vi "Main.vi"(11 "Module Admin":refnum<class "Delacor_lib_QMH_Module Admin.lvclass">) -> ()   [LabVIEW 2020, in "UI.lvlib"]
doc: "This template is based off of the Queued Message Handler design pattern and the Queued Message Handler project template that ships with LabVIEW.\n\nThe main difference is that the queue is private to this module and communication between modules is performed via Broadcast and Request events.\n\nRequest events are wrapped in public API methods and are handled in the Event Handling Loop (EHL) of this VI. Any module can register for Broadcast events sent by this module. The EHL generates messages based on user interface actions.\n\nThe Message Handling Loop (MHL) processes messages generated by the EHL, or by other messages. The messages are string values, so new messages can be added easily to the Message Cases case structure in the MHL. Each message cluster can also provide an optional value for Message Data, which is a variant that can be converted to whatever message-specific data is required.\n_____\nBased on Delacor QMH Project Template 5.0.0.82."
uses:
  UI.lvlib
  <vilib>/Delacor/Delacor QMH/Libraries/Module Admin_class/Delacor_lib_QMH_Module Admin.lvclass
  Module Data--cluster.ctl
  Stop Argument--cluster.ctl
  <vilib>/Delacor/Delacor QMH/Libraries/Message Queue_class/Delacor_lib_QMH_Message Queue.lvclass/Delacor_lib_QMH_Message Queue.ctl
  <vilib>/Utility/miscctls.llb/LVPointTypeDef.ctl
  <vilib>/Delacor/Delacor QMH/Libraries/Module Admin_class/Delacor_lib_QMH_Module Admin.lvclass/Delacor_lib_QMH_Module Admin.ctl
  <vilib>/Delacor/Delacor QMH/Libraries/Message Queue_class/Delacor_lib_QMH_Enqueue Message (Single).vi
  <vilib>/Delacor/Delacor QMH/Libraries/Module Admin_class/Delacor_lib_QMH_Get External Launch.vi
  <vilib>/Utility/error.llb/Error Cluster From Error Code.vi
  <vilib>/ErrorRing/Error Ring.xnode
  <vilib>/Delacor/Delacor QMH/Libraries/Message Queue_class/Delacor_lib_QMH_Message Queue.lvclass
  Acquisition/Acquisition.lvlib
  Config/Config.lvlib
  Loggin/Loggin.lvlib
panel:
  in  "Config":bool
  in  "Stop Acq":bool
  in  "Start Acq":bool
  out "error out":errorcluster
  out "Status":string
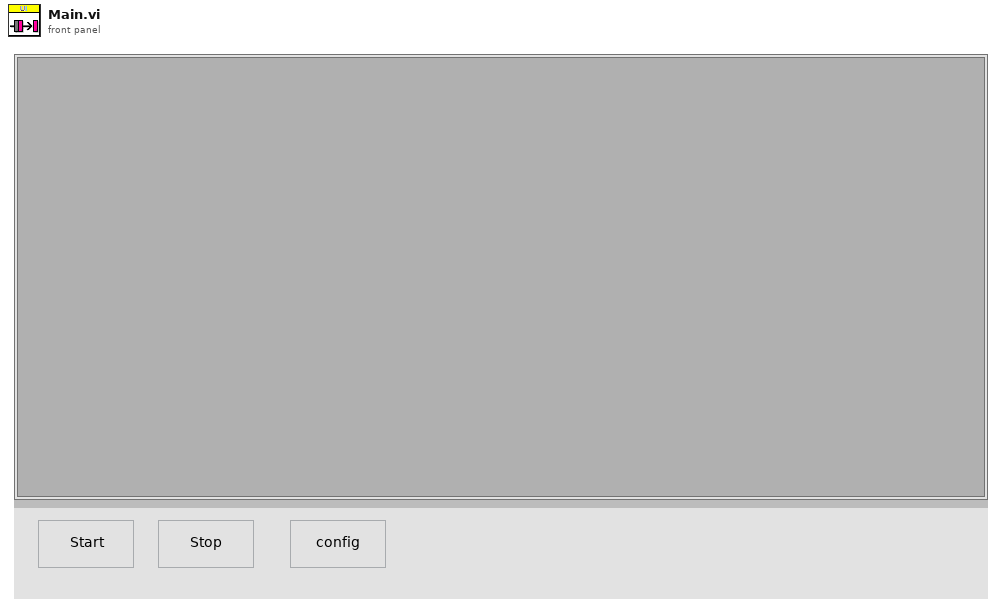
[diagram p1: front panel]
types:
  T1 = typedef "UI.lvlib/Request Events--cluster.ctl" = cluster{"Stop Module":refnum<user-event>, "Show Panel":refnum<user-event>, "Hide Panel":refnum<user-event>, "Get Module Execution Status":refnum<user-event>, "Show Diagram":refnum<user-event>}
  T2 = typedef "Config.lvlib/Broadcast Events--cluster.ctl" = cluster{"Module Did Init":refnum<user-event>, "Status Updated":refnum<user-event>, "Error Reported":refnum<user-event>, "Module Did Stop":refnum<user-event>, "Update Module Execution Status":refnum<user-event>}
  T3 = typedef "Acquisition.lvlib/Broadcast Events--cluster.ctl" = cluster{"Module Did Init":refnum<user-event>, "Status Updated":refnum<user-event>, "Error Reported":refnum<user-event>, "Module Did Stop":refnum<user-event>, "Update Module Execution Status":refnum<user-event>}
  T4 = typedef "Loggin.lvlib/Broadcast Events--cluster.ctl" = cluster{"Module Did Init":refnum<user-event>, "Status Updated":refnum<user-event>, "Error Reported":refnum<user-event>, "Module Did Stop":refnum<user-event>, "Update Module Execution Status":refnum<user-event>}
  T5 = typedef "UI.lvlib/Module Data--cluster.ctl" = cluster{"Status":string}
  T6 = enum32{"invalid lock state", "Not Locked", "Locked (No Password)", "Password-protected"}
  T7 = typedef "UI.lvlib/Stop Argument--cluster.ctl" = cluster{"Origin":string, "Exit via Stop Module Req?":bool, "Wait for Module to stop?":bool}
  T8 = enum32{"Invalid", "Standard", "Closed", "Hidden", "Minimized", "Maximized"}
  T9 = typedef "LVPointTypeDef.ctl" = cluster{"Horizontal":i16, "Vertical":i16}
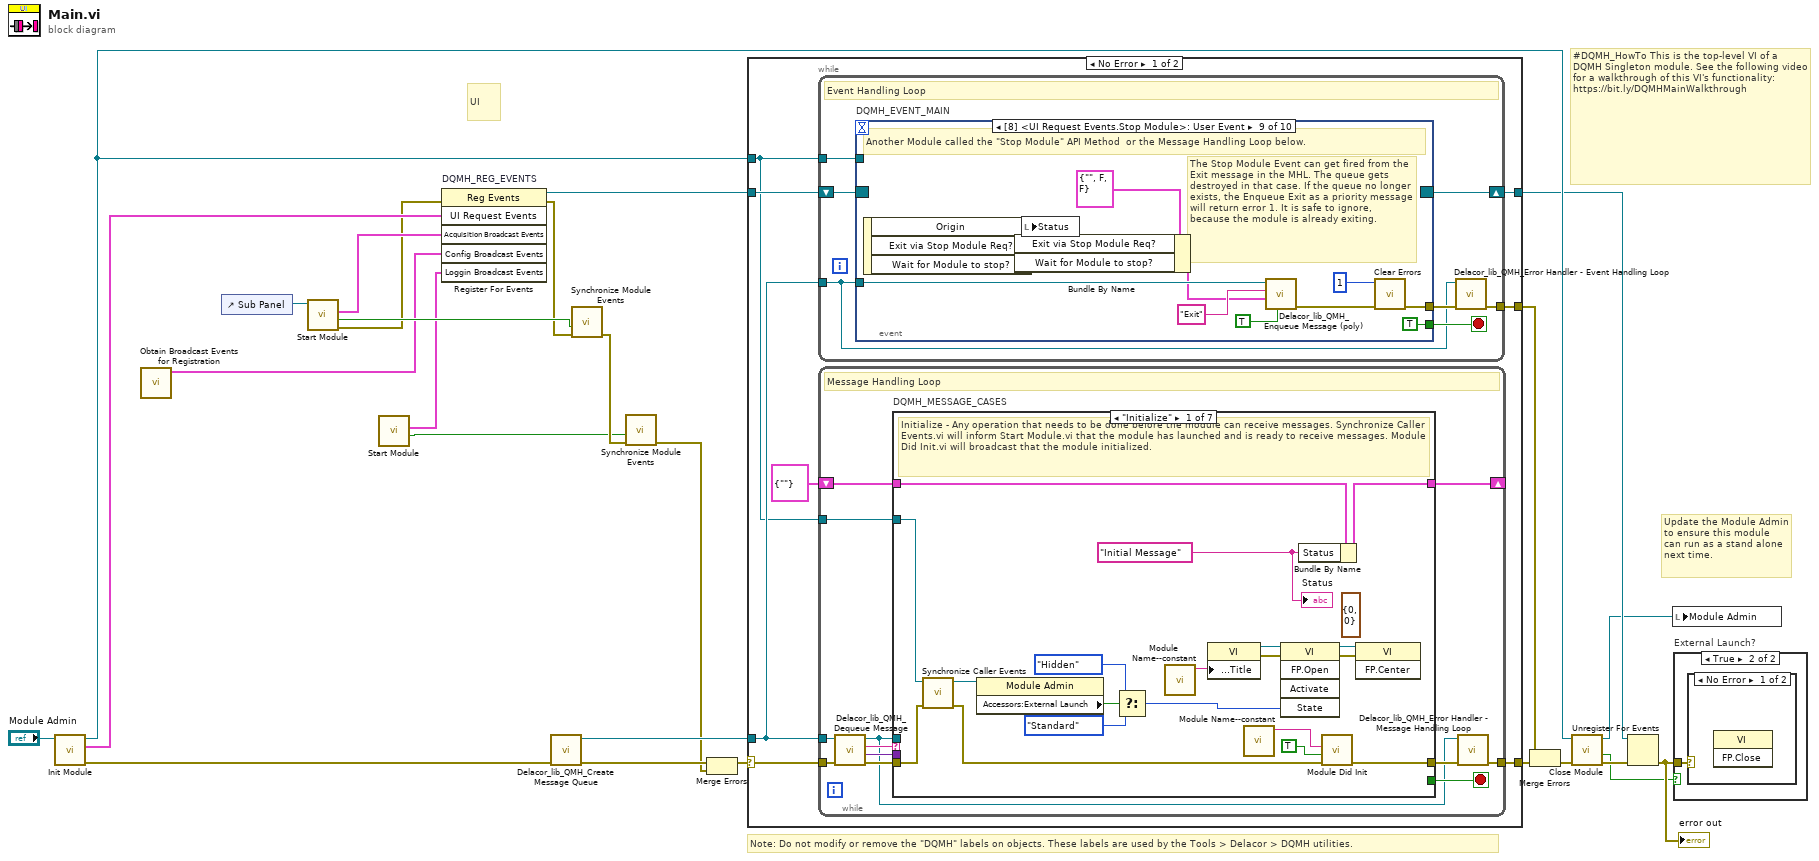
[diagram p0: block diagram]
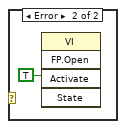
[diagram p3: hidden frame]
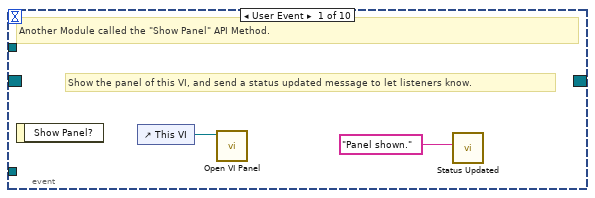
[diagram p4: hidden frame]
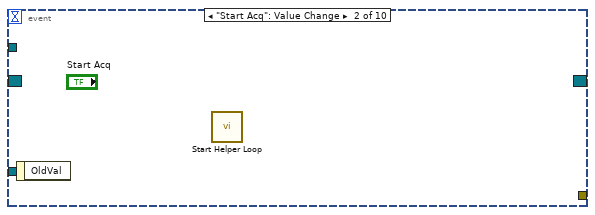
[diagram p5: hidden frame]
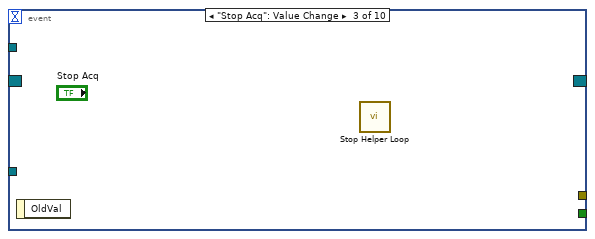
[diagram p6: hidden frame]
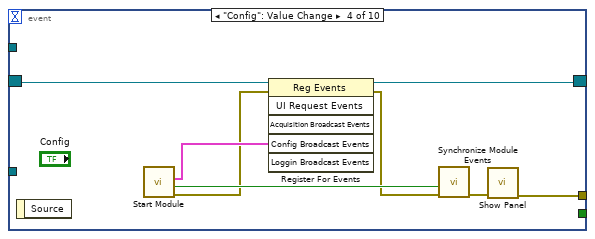
[diagram p7: hidden frame]
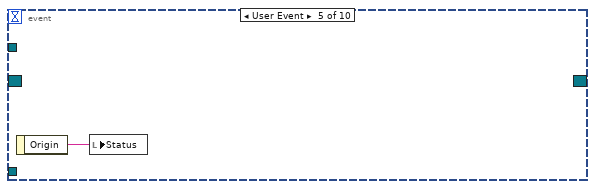
[diagram p8: hidden frame]
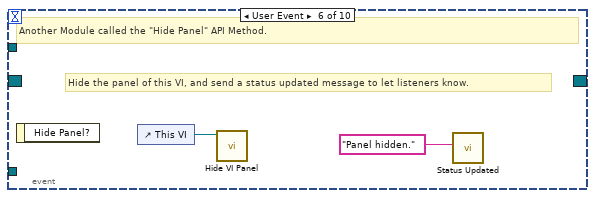
[diagram p9: hidden frame]
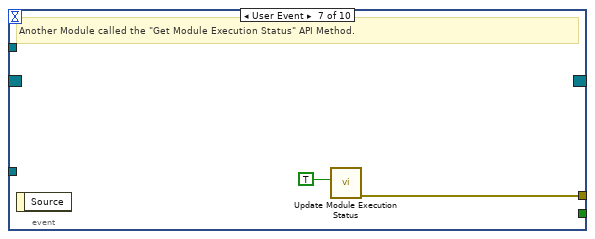
[diagram p10: hidden frame]
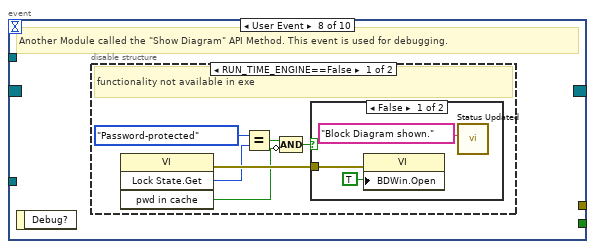
[diagram p11: hidden frame]
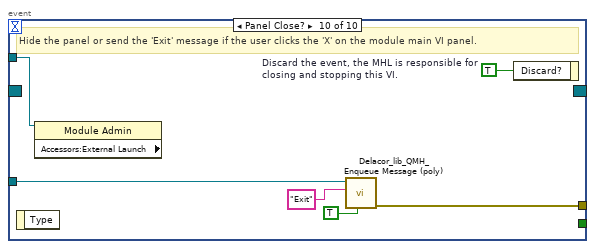
[diagram p14: hidden frame]
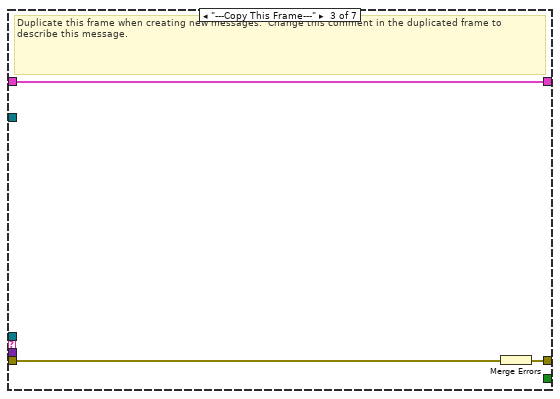
[diagram p16: hidden frame]
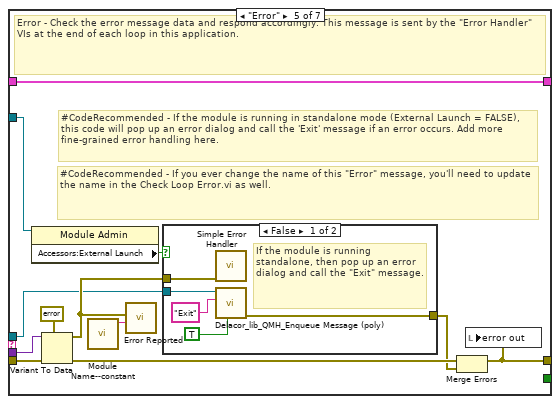
[diagram p18: hidden frame]
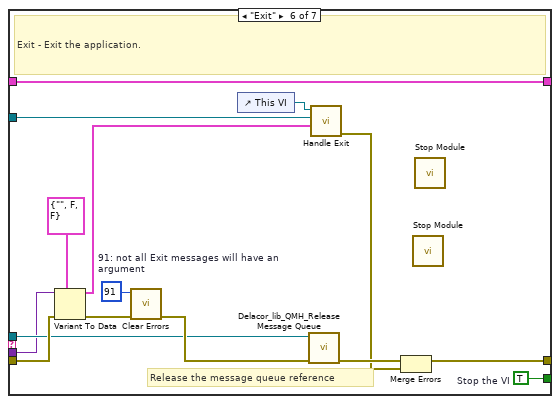
[diagram p20: hidden frame]
diagram:
  # "UI"
  # "#DQMH_HowTo This is the top-level VI of a DQMH Singleton module. See the following video for a walkthrough of this VI's functionality: https://bit.ly/DQMHMainWalkthrough"
  # "Note: Do not modify or remove the \"DQMH\" labels on objects. These labels are used by the Tools > Delacor > DQMH utilities."
  # "Update the Module Admin to ensure this module can run as a stand alone next time."
  n1 = call "Init Module.vi"("Singleton Module Admin in"="Module Admin") -> ("error out"=w25:errorcluster, "UI Request Events"=w15:T1, "Singleton Module Admin out"=w18:refnum<class "Delacor_lib_QMH_Module Admin.lvclass">)  [unwired: 8 in]
  n2 = call "Obtain Broadcast Events for Registration.vi"() -> ("Config Broadcast Events"=w5:T2)  [unwired: 9 in, 2 out]
  n3 = control-ref of="Sub Panel"() -> (w6:refnum<vi>)
  n4 = call "Start Module.vi"("Sub Panel"=w6) -> ("error out"=w7:errorcluster, "Wait for Event Sync?"=w9:bool, "Acquisition Broadcast Events"=w10:T3)  [unwired: 7 in, 1 out]
  n5 = call "Start Module.vi"() -> ("Wait for Event Sync?"=w2:bool, "Loggin Broadcast Events"=w1:T4)  [unwired: 8 in, 2 out]
  n6 = register-events "DQMH_REG_EVENTS"(error in=w7, w15, w10, w5, w1) -> (reference out=w16:refnum<event-registration>, error out=w8:errorcluster)  [unwired: 1 in]
  n7 = call <vilib>:"Delacor_lib_QMH_Create Message Queue.vi"("error in (no error)"=w25) -> ("error out"=w20:errorcluster, "Message Queue"=w14:refnum<class "Delacor_lib_QMH_Message Queue.lvclass">)  [unwired: 9 in]
  n8 = call "Synchronize Module Events.vi"("error in (no error)"=w8, "Wait for Event Sync?"=w9) -> ("error out"=w4:errorcluster)  [unwired: 9 in]
  n9 = call "Synchronize Module Events.vi"("error in (no error)"=w4, "Wait for Event Sync?"=w2) -> ("error out"=w3:errorcluster)  [unwired: 9 in]
  n10 = Merge Errors(w20, w3) -> (w19:errorcluster)
  n11 = case shown="No Error" w19 {
    selector: w19 -> [w32 w170]
    tunnel: [w34 w169] -> w26
    tunnel: [w31 w175] -> w17
    tunnel: w16 -> [w29 w175]
    tunnel: w14 -> [w28 w168]
    tunnel: [w33 _] -> w23
    tunnel: w18 -> [w27 w171]
    frame No Error {
      n12 = while {
        tunnel: w28 -> [w35]
        shift-right: [w38] -> w31
        shift-left: w29 -> [w39]
        tunnel: [w40] -> w33
        tunnel: w27 -> [w36]
        stop <- w37 stop-if-true
        # "Event Handling Loop"
        n13 = event "DQMH_EVENT_MAIN" shown="[8] <UI Request Events.Stop Module>: User Event" {
          selector: w39 -> [_ _ _ w51 _ _ _ _ _ _]
          dyn-events: [_ _ _ w50 _ _ _ _ _ _] -> w38
          timeout: _ -> [_ _ _ _ _ _ _ _ _ _]
          tunnel: [_ _ _ _ _ _ _ _ TRUE ("Discard?") _] -> w37
          tunnel: w35 -> [_ _ _ _ _ _ _ _ w73 w81]
          tunnel: [_ _ _ w44 _ _ w56 _ w76 w83] -> w41
          tunnel: w36 -> [_ _ _ _ _ _ _ _ _ w80]
          event User Event {
            # "Show the panel of this VI, and send a status updated message to let listeners know."
            # "Another Module called the \"Show Panel\" API Method."
            n14 = event-data() -> ()  [unwired: 1 in, 1 out]
            n15 = control-ref of="This VI"() -> (w43:refnum<vi>)
            n16 = call "Open VI Panel.vi"("VI"=w43) -> ()  [unwired: 10 in, 1 out]
            n17 = call "Status Updated.vi"("Status"="Panel shown." ("format string")) -> ()  [unwired: 10 in, 1 out]
          }
          event "Start Acq": Value Change {
            n18 = event-data() -> ()  [unwired: 1 in, 1 out]
            n19 = call "Start Helper Loop.vi"() -> ()  [unwired: 11 in, 1 out]
          }
          event "Stop Acq": Value Change {
            n20 = event-data() -> ()  [unwired: 1 in, 1 out]
            n21 = call "Stop Helper Loop.vi"() -> ()  [unwired: 11 in, 1 out]
          }
          event "Config": Value Change {
            n22 = event-data() -> ()  [unwired: 1 in, 1 out]
            n23 = call "Start Module.vi"() -> ("error out"=w47:errorcluster, "Wait for Event Sync?"=w48:bool, "Config Broadcast Events"=w49:T2)  [unwired: 8 in, 1 out]
            n24 = register-events(reference=w51, error in=w47, w49) -> (reference out=w50:refnum<event-registration>, error out=w46:errorcluster)  [unwired: 3 in]
            n25 = call "Synchronize Module Events.vi"("error in (no error)"=w46, "Wait for Event Sync?"=w48) -> ("error out"=w45:errorcluster)  [unwired: 9 in]
            n26 = call "Show Panel.vi"("error in (no error)"=w45) -> ("error out"=w44:errorcluster)  [unwired: 10 in]
          }
          event User Event {
            n27 = event-data() -> ("Origin"=w52:string)  [unwired: 1 in]
            n28 = local write "Status"(w52) -> ()
          }
          event User Event {
            # "Hide the panel of this VI, and send a status updated message to let listeners know."
            # "Another Module called the \"Hide Panel\" API Method."
            n29 = event-data() -> ()  [unwired: 1 in, 1 out]
            n30 = control-ref of="This VI"() -> (w54:refnum<vi>)
            n31 = call "Hide VI Panel.vi"("VI"=w54) -> ()  [unwired: 10 in, 1 out]
            n32 = call "Status Updated.vi"("Status"="Panel hidden." ("format string")) -> ()  [unwired: 10 in, 1 out]
          }
          event User Event {
            # "Another Module called the \"Get Module Execution Status\" API Method."
            n33 = event-data() -> ()  [unwired: 1 in, 1 out]
            n34 = call "Update Module Execution Status.vi"("Running?"=TRUE) -> ("error out"=w56:errorcluster)  [unwired: 10 in]
          }
          event User Event {
            # "Another Module called the \"Show Diagram\" API Method. This event is used for debugging."
            n35 = event-data() -> ()  [unwired: 1 in, 1 out]
            n36 = disable-structure shown="RUN_TIME_ENGINE==False" {
              frame condition #0 (active) {
                # "functionality not available in exe"
                n37 = invoke class="VI" method="Lock State.Get"() -> (error out=w62:errorcluster, "Get Lock State"=w61:T6, "pwd in cache"=w58:bool)  [unwired: 4 in, 1 out]
                n38 = Equal?(x=T6."Password-protected", y=w61) -> (x = y?=w59:bool)
                n39 = Compound Arithmetic op=AND(w59, invert w58) -> (w57:bool)
                n40 = case shown="False" w57 {
                  tunnel: w62 -> [w65 _]
                  frame False {
                    n41 = property class="VI"(error in=w65, "BDWin.Open"=TRUE ("Block Diagram Window:Open")) -> ()  [unwired: 1 in, 2 out]
                    n42 = call "Status Updated.vi"("Status"="Block Diagram shown." ("format string")) -> ()  [unwired: 10 in, 1 out]
                  }
                  frame True {
                    # "Password-protected VI, and the password is not in the cache. Do not show the diagram."
                  }
                }
              }
              frame condition #1 {
              }
            }
          }
          event User Event {
            # "The Stop Module Event can get fired from the Exit message in the MHL. The queue gets destroyed in that case. If the queue no longer exists, the Enqueue Exit as a priority message will return error 1. It is safe to ignore, because the module is already exiting."
            # "Another Module called the \"Stop Module\" API Method  or the Message Handling Loop below."
            n43 = event-data() -> ("Origin"=w72:string, "Exit via Stop Module Req?"=w68:bool, "Wait for Module to stop?"=w67:bool)  [unwired: 1 in]
            n44 = Bundle By Name(cluster=T7 {"Origin"="", "Exit via Stop Module Req?"=FALSE, "Wait for Module to stop?"=FALSE} ("Stop Argument"), "Exit via Stop Module Req?"=w68, "Wait for Module to stop?"=w67) -> (w66:T7)
            n45 = local write "Status"(w72) -> ()
            n46 = call-poly <vilib>:"Delacor_lib_QMH_Enqueue Message (poly).vi"("Priority Message? (F)"=TRUE, "Message Data"=w66, "Message"="Exit", "Message Queue in"=w73) -> ("error out"=w77:errorcluster)  [unwired: 6 in, 1 out]
            n47 = call <vilib>:"Clear Errors.vi"("error in (no error)"=w77, "specific error code to clear (0: all)"=1) -> ("error out"=w76:errorcluster)  [unwired: 4 in, 1 out]
          }
          event Panel Close? {
            w82 = TRUE  # Discard the event, the MHL is responsible for closing and stopping this VI.
            # "Hide the panel or send the 'Exit' message if the user clicks the 'X' on the module main VI panel."
            n48 = event-data() -> ()  [unwired: 1 in, 1 out]
            n49 = property class="Module Admin" props=["Accessors:External Launch"](reference=w80) -> ()  [unwired: 1 in, 3 out]
            n50 = call-poly <vilib>:"Delacor_lib_QMH_Enqueue Message (poly).vi"("Priority Message? (F)"=TRUE, "Message"="Exit", "Message Queue in"=w81) -> ("error out"=w83:errorcluster)  [unwired: 7 in, 1 out]
            n51 = event-data("Discard?"=w82) -> ()  [unwired: 1 in, 1 out]
          }
        }
        n52 = call-dynamic "Delacor_lib_QMH_Error Handler - Event Handling Loop.vi"("error in (no error)"=w41, "Message Queue in"=w35) -> ("dup error in"=w40:errorcluster)  [unwired: 8 in, 1 out]
      }
      n53 = while {
        tunnel: w28 -> [w86]
        shift-right: [w90] -> _
        shift-left: T5 {"Status"=""} ("Data Cluster") -> [w91]
        tunnel: w32 -> [w94]
        tunnel: [w92] -> w34
        tunnel: w27 -> [w84]
        stop <- w89 stop-if-true
        # "Message Handling Loop"
        n54 = call-dynamic "Delacor_lib_QMH_Dequeue Message.vi"("error in (no error)"=w94, "Message Queue in"=w86) -> ("error out"=w93:errorcluster, "Message Data"=w87:variant, "Message"=w88:string, "Message Queue out"=w85:refnum<class "Delacor_lib_QMH_Message Queue.lvclass">)  [unwired: 6 in]
        n55 = case "DQMH_MESSAGE_CASES" shown="\"Initialize\"" w88 {
          selector: w88 -> [_ _ _ _ _ _ w155]
          tunnel: w85 -> [_ _ _ _ w125 w147 _]
          tunnel: w93 -> [w112 w116 w119 w121 w132 w153 w157]
          tunnel: [w110 w116 w118 w121 w128 w150 w158] -> w95
          tunnel: w91 -> [w101 w115 w117 w120 w127 w146 w156]
          tunnel: [w100 w115 w117 w120 w127 w146 w156] -> w90
          tunnel: [_ _ _ _ _ w145 _] -> w89
          tunnel: w87 -> [_ _ _ _ w126 w144 _]
          tunnel: w84 -> [w102 _ _ _ w124 w139 _]
          frame "Initialize" {
            (unwired) T9 {"Horizontal"=0, "Vertical"=0} ("Origin")
            w96 = "Initial Message" ("Initial Message")
            # "Initialize - Any operation that needs to be done before the module can receive messages. Synchronize Caller Events.vi will inform Start Module.vi that the module has launched and is ready to receive messages. Module Did Init.vi will broadcast that the module initialized."
            n56 = call "Synchronize Caller Events.vi"("error in (no error)"=w112, "Singleton Module Admin in"=w102) -> ("error out"=w111:errorcluster, "Singleton Module Admin out"=w97:refnum<class "Delacor_lib_QMH_Module Admin.lvclass">)  [unwired: 8 in]
            n57 = property class="Module Admin"(reference=w97) -> ("Accessors:External Launch"=w106:bool)  [unwired: 1 in, 2 out]
            n58 = Select(t=T8."Hidden" ("State"), s=w106, f=T8."Standard" ("State")) -> (s? t:f=w103:T8)
            n59 = call "Module Name--constant.vi"() -> ("Module Name"=w109:string)  [unwired: 11 in]
            n60 = property class="VI"("Front Panel.Title"=w109) -> (reference out=w108:refnum<vi>, error out=w114:errorcluster)  [unwired: 2 in]
            n61 = call "Module Name--constant.vi"() -> ("Module Name"=w98:string)  [unwired: 11 in]
            n62 = invoke class="VI" method="FP.Open"(reference=w108, error in=w114, "State"=w103) -> (reference out=w107:refnum<vi>, error out=w113:errorcluster)  [unwired: 2 in, 3 out]
            n63 = Bundle By Name(cluster=w101, "Status"=w96) -> (w100:T5)
            n64 = call "Module Did Init.vi"("error in (no error)"=w111, "Initialized?"=TRUE, "Origin"=w98) -> ("error out"=w110:errorcluster)  [unwired: 8 in]
            n65 = invoke class="VI" method="FP.Center"(reference=w107, error in=w113) -> ()  [unwired: 1 in, 3 out]
            "Status" <- w96
          }
          frame "--- Module Specific ---" {
            # "Separator -- The following cases handle messages specific to this Module."
          }
          frame "---Copy This Frame---" {
            # "Duplicate this frame when creating new messages.  Change this comment in the duplicated frame to describe this message."
            n66 = Merge Errors(w119) -> (w118:errorcluster)
          }
          frame "--- Exit and Error Handling---" {
            # "Separator - The following cases handle errors and exit messages."
          }
          frame "Error" {
            # "#CodeRecommended - If you ever change the name of this \"Error\" message, you'll need to update the name in the Check Loop Error.vi as well."
            # "#CodeRecommended - If the module is running in standalone mode (External Launch = FALSE), this code will pop up an error dialog and call the 'Exit' message if an error occurs. Add more fine-grained error handling here."
            # "Error - Check the error message data and respond accordingly. This message is sent by the \"Error Handler\" VIs at the end of each loop in this application."
            n67 = property class="Module Admin"(reference=w124) -> ("Accessors:External Launch"=w123:bool)  [unwired: 1 in, 2 out]
            n68 = Variant To Data(error in=w132, type=errorcluster {"status"=FALSE, "code"=0, "source"=""} ("error constant"), Variant=w126) -> (data=w133:errorcluster, error out=w130:errorcluster)
            n69 = call "Module Name--constant.vi"() -> ("Module Name"=w122:string)  [unwired: 11 in]
            n70 = call "Error Reported.vi"("Additional Information"=w122, "Error"=w133) -> ()  [unwired: 9 in, 1 out]
            n71 = case shown="False" w123 {
              tunnel: [w138 _] -> w129
              tunnel: w125 -> [w136 _]
              tunnel: w133 -> [w137 _]
              frame False {
                # "If the module is running standalone, then pop up an error dialog and call the \"Exit\" message."
                n72 = call <vilib>:"Simple Error Handler.vi"("error in (no error)"=w137) -> ()  [unwired: 4 in, 5 out]
                n73 = call-poly <vilib>:"Delacor_lib_QMH_Enqueue Message (poly).vi"("Priority Message? (F)"=TRUE, "Message"="Exit", "Message Queue in"=w136) -> ("error out"=w138:errorcluster)  [unwired: 7 in, 1 out]
              }
              frame True {
                # "If the module was launched externally, calling the Error Reported broadcast VI is the only action performed by the \"Error\" message. The module's caller can then process the error appropriately."
              }
            }
            n74 = Merge Errors(w130, w129) -> (w128:errorcluster)
            n75 = local write "error out"(w128) -> ()
          }
          frame "Exit" {
            w143 = 91  # 91: not all Exit messages will have an argument
            w145 = TRUE  # Stop the VI
            # "Release the message queue reference"
            # "Exit - Exit the application."
            n76 = Variant To Data(error in=w153, type=T7 {"Origin"="", "Exit via Stop Module Req?"=FALSE, "Wait for Module to stop?"=FALSE} ("Stop Argument"), Variant=w144) -> (data=w141:T7, error out=w149:errorcluster)
            n77 = call <vilib>:"Clear Errors.vi"("error in (no error)"=w149, "specific error code to clear (0: all)"=w143) -> ("error out"=w152:errorcluster)  [unwired: 4 in, 1 out]
            n78 = control-ref of="This VI"() -> (w140:refnum<vi>)
            n79 = call-dynamic "Delacor_lib_QMH_Release Message Queue.vi"("error in (no error)"=w152, "Message Queue"=w147) -> ("error out"=w151:errorcluster)  [unwired: 9 in]
            n80 = call "Handle Exit.vi"("Stop Argument"=w141, "Admin in"=w139, "VI reference"=w140) -> ("error out"=w148:errorcluster)  [unwired: 7 in, 1 out]
            n81 = Merge Errors(w151, w148) -> (w150:errorcluster)
            n82 = call "Stop Module.vi"() -> ()  [unwired: 11 in, 1 out]
            n83 = call "Stop Module.vi"() -> ()  [unwired: 11 in, 1 out]
          }
          frame Default {
            # "'Default' case only runs if there is a message that isn't defined in any of the other cases.  Output a programming error."
            n84 = call "Module Name--constant.vi"() -> ("Module Name"=w154:string)  [unwired: 11 in]
            n85 = xnode "Error Ring"("parameter 0"=w155, "parameter 1"=w154) -> ("error out"=w159:errorcluster)
            n86 = Merge Errors(w157, w159) -> (w158:errorcluster)
          }
        }
        n87 = call-dynamic "Delacor_lib_QMH_Error Handler - Message Handling Loop.vi"("error in (no error)"=w95, "Message Queue in"=w85) -> ("dup error in"=w92:errorcluster)  [unwired: 8 in, 1 out]
      }
    }
    frame Error {
      # "Synchronize Caller Events.vi will inform Start Module.vi that the module has launched and will let the code calling Start Module.vi register for broadcasts and would permit the caller receive the broadcast that an error occurred at launch time."
      n88 = call-dynamic "Delacor_lib_QMH_Release Message Queue.vi"("error in (no error)"=w170, "Message Queue"=w168) -> ("error out"=w169:errorcluster)  [unwired: 9 in]
      n89 = call "Synchronize Caller Events.vi"("Singleton Module Admin in"=w171) -> ("error out"=w176:errorcluster)  [unwired: 9 in, 1 out]
      n90 = call "Module Name--constant.vi"() -> ("Module Name"=w174:string)  [unwired: 11 in]
      n91 = Format Into String(format string="An error occurred during initialization. %s is no longer running.", w174) -> (resulting string=w172:string)  [unwired: 2 in, 1 out]
      n92 = Merge Errors(w169, w176) -> (w177:errorcluster)
      n93 = call "Error Reported.vi"("Additional Information"=w172, "Error"=w177) -> ()  [unwired: 9 in, 1 out]
    }
  }
  n94 = Merge Errors(w23, w26) -> (w22:errorcluster)
  n95 = call "Close Module.vi"("error in (no error)"=w22, "Module Admin in"=w18) -> ("error out"=w24:errorcluster, "External Launch"=w11:bool, "Module Admin out"=w12:refnum<class "Delacor_lib_QMH_Module Admin.lvclass">)  [unwired: 7 in]
  n96 = Unregister For Events(event registration refnum=w17, error in=w24) -> (error out=w21:errorcluster)
  "error out" <- w21
  n97 = local write "Module Admin"(w12) -> ()
  n98 = case "External Launch?" shown="True" w11 {
    tunnel: w21 -> [_ w178]
    frame False {
    }
    frame True {
      n99 = case shown="No Error" w178 {
        frame No Error {
          n100 = invoke class="VI" method="FP.Close"() -> ()  [unwired: 3 in, 3 out]
        }
        frame Error {
          n101 = invoke class="VI" method="FP.Open"("Activate"=TRUE ("Activate?")) -> ()  [unwired: 4 in, 5 out]
        }
      }
    }
  }
